vi "Tests.vi"() -> ()   [LabVIEW 2012]
uses:
  <vilib>/Analysis/NI_AALBase.lvlib
panel:
  out "ErrorOut 5":errorcluster
  out "ErrorOut 4":errorcluster
  out "ErrorOut 3":errorcluster
  out "ErrorOut 2":errorcluster
  out "ErrorOut":errorcluster
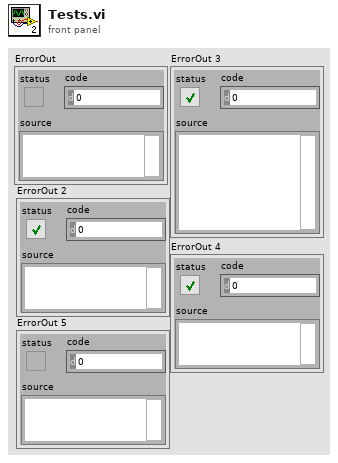
[diagram p1: front panel]
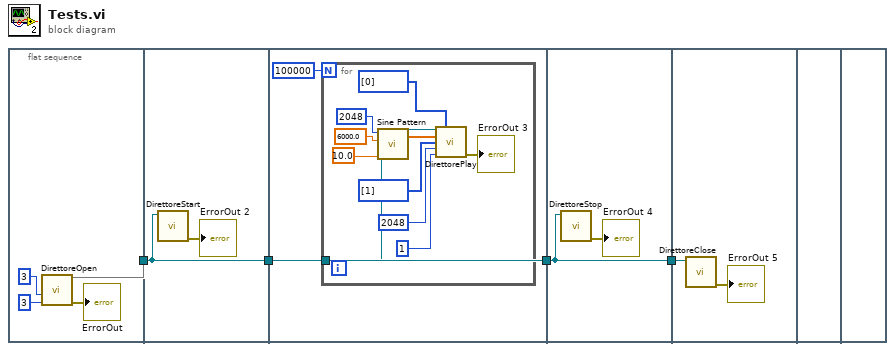
[diagram p0: block diagram]
diagram:
  n1 = flat-sequence {
    tunnel: [w5] -> w1
    tunnel: [w9] -> w4
    tunnel: w1 -> [w9]
    tunnel: w4 -> [w12]
    tunnel: [w12] -> w3
    tunnel: w3 -> [w23]
    tunnel: [w23] -> w2
    tunnel: w2 -> [w25]
    frame #0 {
      n2 = call "DirettoreOpen.vi"("MatrixFIFODepth"=3, "TriggerFIFODepth"=u32 3) -> ("ErrorOut"=→"ErrorOut":errorcluster, 11:w5)  [unwired: 7 in, 1 out]
    }
    frame #1 {
      n3 = call "DirettoreStart.vi"("FPGAReference"=w9) -> ("ErrorOut"=→"ErrorOut 2":errorcluster)  [unwired: 10 in]
    }
    frame #2 {
      n4 = for {
        N: 100000 -> [_]
        tunnel: w12 -> [w21]
        n5 = call <vilib>:"Sine Pattern.vi"("cycles"=10.0, "amplitude"=6000.0, "samples"=2048) -> ("Sinusoidal Pattern"=w19:dbl[])  [unwired: 1 in, 1 out]
        n6 = call "DirettorePlay.vi"("FPGAReference"=w21, "Sync"=i16[] [0], "MatricesArray"=w19, "DeltaTimeArray"=i16[] [1], "NumberOfTimePointsToPlay"=u32 2048, "NumberOfMatrices"=u32 1) -> ("ErrorOut"=→"ErrorOut 3":errorcluster)  [unwired: 8 in, 1 out]
      }
    }
    frame #3 {
      n7 = call "DirettoreStop.vi"("FPGAReference"=w23) -> ("ErrorOut"=→"ErrorOut 4":errorcluster)  [unwired: 10 in]
    }
    frame #4 {
      n8 = call "DirettoreClose.vi"("FPGAReference"=w25) -> ("ErrorOut"=→"ErrorOut 5":errorcluster)  [unwired: 10 in]
    }
    frame #5 {
    }
    frame #6 {
    }
  }
